vi "class_data.vi"() -> ()   [LabVIEW 2010, in "GenericExperimentController.lvclass"]
uses:
  GenericExperimentController.lvclass
panel:
  in  "latest instance":refnum<class "GenericExperimentController.lvclass">
  in  "locked by":string
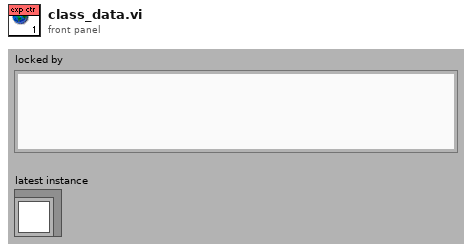
[diagram p1: front panel]
diagram:
